vi "Test Read Linker Info.vi"(8 "error in (no error)":errorcluster) -> (0 "error out":errorcluster)   [LabVIEW 2013]
uses:
  classes/Test Runner/Test Runner.lvclass
  classes/Test/Test.lvclass
  classes/Assert/Assert.lvclass
panel:
  out "Test VIs":path[](array[path])
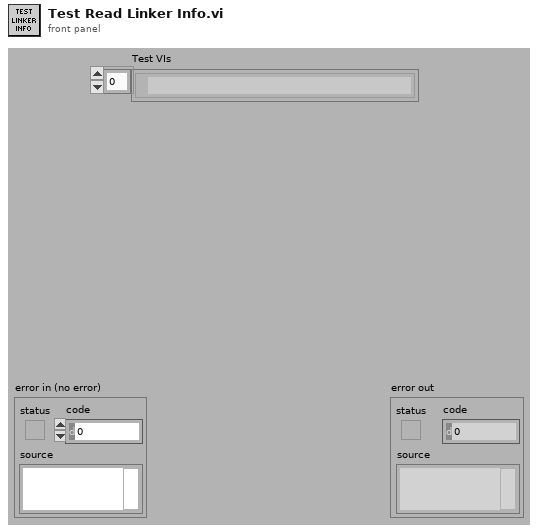
[diagram p1: front panel]
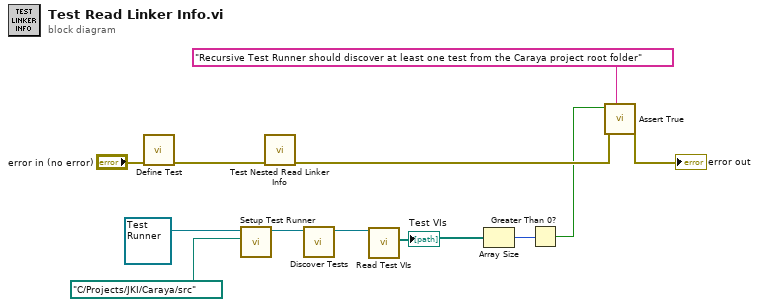
[diagram p0: block diagram]
diagram:
  n1 = call "Define Test.vi"("error in (no error)"="error in (no error)") -> ("error out"=w11:errorcluster)  [unwired: 10 in]
  n2 = call "Setup Test Runner.vi"("Directory to search"=path "C:/Projects/JKI/Caraya/src", "Test Runner in"=refnum<class "Test Runner.lvclass"> refnum ("Caraya.lvlib:Test Runner.lvclass")) -> ("Test Runner out"=w8:refnum<class "Test Runner.lvclass">)  [unwired: 8 in, 1 out]
  n3 = call "Test Nested Read Linker Info.vi"("error in (no error)"=w11) -> ("error out"=w4:errorcluster)  [unwired: 10 in]
  n4 = call-dynamic "Discover Tests.vi"("Test Runner in"=w8) -> ("Test Runner out"=w7:refnum<class "Test Runner.lvclass">)  [unwired: 9 in, 1 out]
  n5 = call-dynamic "Read Test VIs.vi"("Test Runner in"=w7) -> ("Test VIs"=w6:path[])  [unwired: 8 in, 2 out]
  "Test VIs" <- w6
  n6 = Array Size(array=w6) -> (size(s)=w5:i32)
  n7 = Greater Than 0?(x=w5) -> (x > 0?=w2:bool)
  n8 = call "Assert True.vi"("Label"="Recursive Test Runner should discover at least one test from the Caraya project root folder", "error in (no error)"=w4, "True?"=w2) -> ("error out"=→"error out":errorcluster)  [unwired: 8 in]
